vi "M02 Toy Factory - Dahai.vi"(11 "EV3 in":T1) -> (3 "NXT/EV3":T1)   [LabVIEW 2016]
uses:
  <vilib>/NXT/Subs/LVHSConnector.ctl
  <vilib>/NXT/LegoClasses/BrickReference/BrickReference.lvclass
  <vilib>/NXT/Block Support/NXT_OutputPort.ctl
  <vilib>/NXT/NXTIO Xnodes/NXTIONodeSubVIs/NXTMotorRunDistance.vi
  <vilib>/NXT/Dual Mode Library/Waits/Wait_Num(msec).vi
  <vilib>/NXT/NXTIO Xnodes/AddressXNode/NXTIOAddress.xnode
  <vilib>/NXT/NXTIO Xnodes/NXTIOXNode/NXTIO.xnode
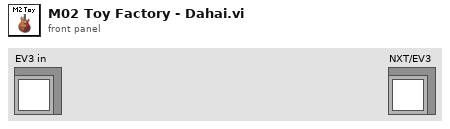
[diagram p1: front panel]
types:
  T1 = typedef "LVHSConnector.ctl" = refnum<class "BrickReference.lvclass">
  T2 = typedef "NXT_OutputPort.ctl" = u8
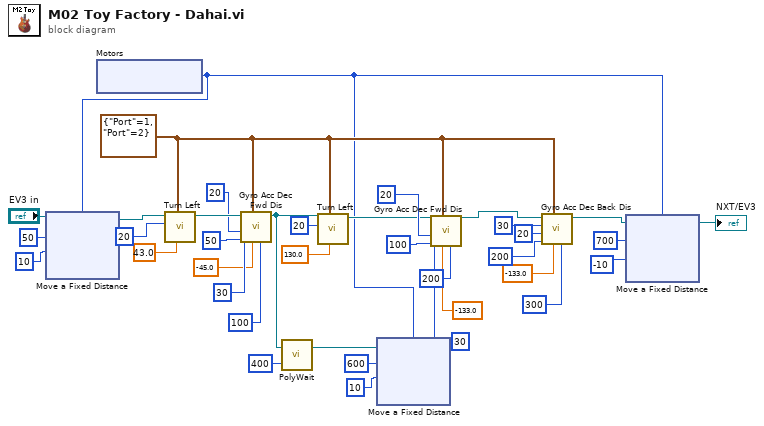
[diagram p0: block diagram]
diagram:
  w13 = cluster{"Port":T2, "Port":T2} {"Port"=1, "Port"=2} ("Motor")
  n1 = xnode "Motors"() -> ("Motor"=w1:T2)
  n2 = xnode "Move a Fixed Distance"("Speed 1"=i8 10, "Distance 1"=50, "Motors"=w1, "NXT/EV3"="EV3 in") -> ("NXT/EV3"=w2:T1)
  n3 = call "Turn Left.vi"("Turning angle"=sgl 43.0, "Motor"=w13, "Motor B (right)"=i8 20, "EV3 in"=w2) -> ("EV3 out"=w20:T1)  [unwired: 7 in]
  n4 = call "Gyro Acc Dec Fwd Dis.vi"("Stop rotation"=100, "Ini. Degrees"=sgl -45.0, "Motor"=w13, "Threshold to De-acc"=50, "De-acc"=20, "Acc"=30, "EV3 in"=w20) -> ("EV3 out"=w6:T1)  [unwired: 4 in]
  n5 = call-poly <vilib>:"PolyWait.vi"("Time (100 msec)"=u32 400, "NXT/EV3"=w6) -> ("NXT/EV3"=w9:T1)  [unwired: 2 in]
  n6 = call "Turn Left.vi"("Turning angle"=sgl 130.0, "Motor"=w13, "Motor B (right)"=i8 20, "EV3 in"=w6) -> ("EV3 out"=w7:T1)  [unwired: 7 in]
  n7 = xnode "Move a Fixed Distance"("Speed 1"=i8 10, "Distance 1"=600, "Motors"=w1, "NXT/EV3"=w9) -> ()  [unwired: 1 out]
  n8 = call "Gyro Acc Dec Fwd Dis.vi"("Stop rotation"=200, "Ini. Degrees"=sgl -133.0, "Motor"=w13, "Threshold to De-acc"=100, "De-acc"=20, "Acc"=30, "EV3 in"=w7) -> ("EV3 out"=w34:T1)  [unwired: 4 in]
  n9 = call "Gyro Acc Dec Back Dis.vi"("Stop rotation"=300, "Ini. Degrees"=sgl -133.0, "Motor"=w13, "Threshold to De-acc"=200, "De-acc"=20, "Acc"=30, "EV3 in"=w34) -> ("EV3 out"=w37:T1)  [unwired: 4 in]
  n10 = xnode "Move a Fixed Distance"("Speed 1"=i8 -10, "Distance 1"=700, "Motors"=w1, "NXT/EV3"=w37) -> ("NXT/EV3"=→"NXT/EV3":T1)
